vi "F5xxx Config Panel.vi"(8 "error in":errorcluster, 11 "session in":T2) -> (0 "error out":errorcluster, 3 "session out":T2)   [LabVIEW 2020]
doc: "Fluke 5000 series calibrators configuration panel."
uses:
  F5xxx_session.ctl
  F5xxx_output_mode.ctl
  <vilib>/Utility/error.llb/DialogType.ctl
panel:
  in  "btn test":bool caption="OK Button"
  out "idn string":string caption="Identification string"
  in  "btn ok":bool caption="OK Button"
  in  "ext ref clk":bool
  in  "earth":bool
  in  "mode":T1 caption="Output mode"
  in  "VISA":refnum<visa-resource-name> caption="VISA address"
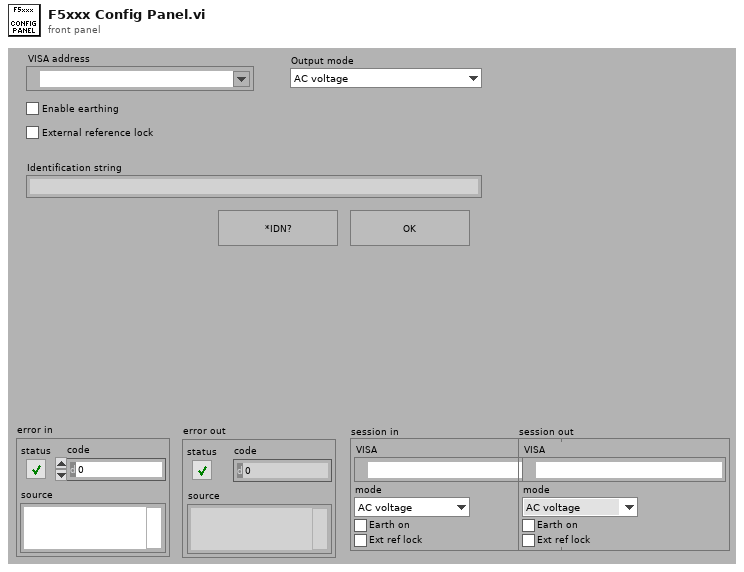
[diagram p1: front panel]
types:
  T1 = typedef "F5xxx_output_mode.ctl" = enum16{"AC voltage", "AC current"}
  T2 = typedef "F5xxx_session.ctl" = cluster{"VISA":refnum<visa-resource-name>, "mode":T1, "Earth on":bool, "Ext ref lock":bool}
  T3 = typedef "DialogType.ctl" = u16
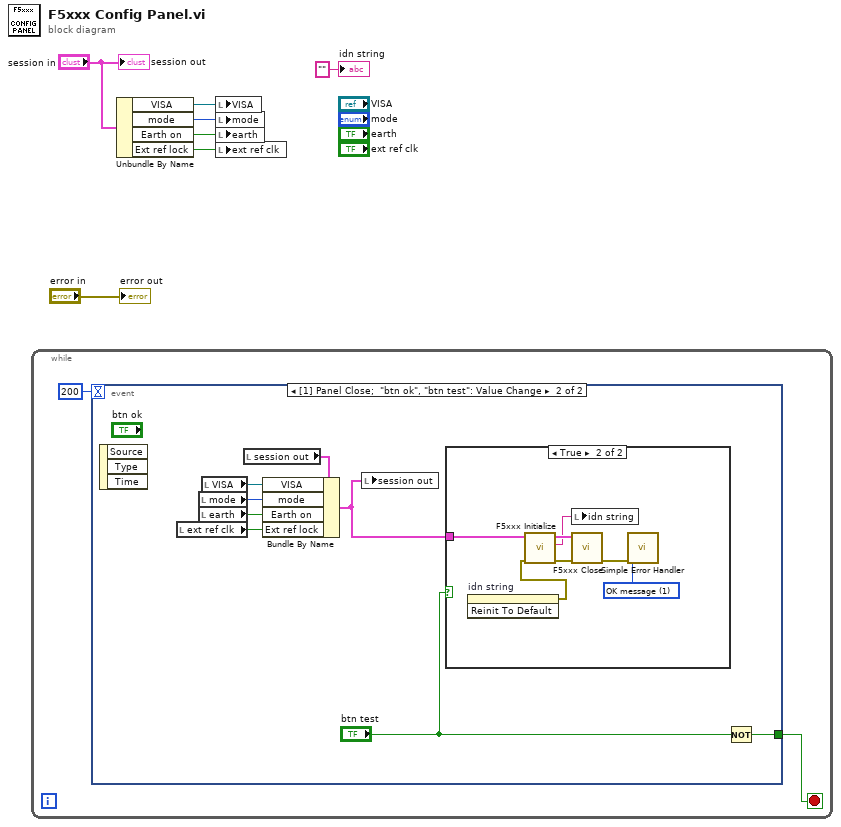
[diagram p0: block diagram]
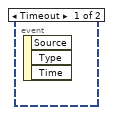
[diagram p2: hidden frame]
diagram:
  n1 = while {
    stop <- w9 stop-if-true
    n2 = event shown="[1] Panel Close;  \"btn ok\", \"btn test\": Value Change" {
      selector: _ -> [_ _]
      dyn-events: _ -> [_ _]
      timeout: 200 -> [_ _]
      tunnel: [_ w12] -> w9
      event Timeout {
        n3 = event-data() -> ()  [unwired: 1 in, 3 out]
      }
      event Panel Close; "btn ok", "btn test": Value Change {
        n4 = event-data() -> ()  [unwired: 1 in, 3 out]
        n5 = local read "ext ref clk"() -> (w13:bool)
        n6 = local read "mode"() -> (w15:T1)
        n7 = local read "earth"() -> (w14:bool)
        n8 = local read "VISA"() -> (w16:refnum<visa-resource-name>)
        n9 = local read "session out"() -> (w17:T2)
        n10 = Bundle By Name(cluster=w17, "VISA"=w16, "mode"=w15, "Earth on"=w14, "Ext ref lock"=w13) -> (w11:T2)
        n11 = local write "session out"(w11) -> ()
        n12 = case shown="True" "btn test" {
          tunnel: w11 -> [_ w24]
          frame False {
          }
          frame True {
            w20 = T3 1 items=["no dialog", "OK message", "continue or stop message", "OK message + warnings", "continue/stop + warnings"] ("type of dialog (OK msg:1)")
            n13 = invoke on="idn string" class="Str" method="Reinit To Default"() -> (error out=w19:errorcluster)  [unwired: 3 in, 2 out]
            n14 = call "F5xxx Initialize.vi"("error in (no error)"=w19, "session in"=w24) -> ("error out"=w23:errorcluster, "idn string"=w18:string, "session out"=w22:T2)  [unwired: 7 in]
            n15 = local write "idn string"(w18) -> ()
            n16 = call "F5xxx Close.vi"("error in (no error)"=w23, "session in"=w22) -> ("error out"=w21:errorcluster)  [unwired: 8 in, 1 out]
            n17 = call <vilib>:"Simple Error Handler.vi"("type of dialog (OK msg:1)"=w20, "error in (no error)"=w21) -> ()  [unwired: 3 in, 5 out]
          }
        }
        n18 = Not(x="btn test") -> (.not. x?=w12:bool)
      }
    }
  }
  n19 = Unbundle By Name("session in") -> ("VISA"=w5:refnum<visa-resource-name>, "mode"=w4:T1, "Earth on"=w3:bool, "Ext ref lock"=w2:bool)
  n20 = local write "VISA"(w5) -> ()
  n21 = local write "mode"(w4) -> ()
  n22 = local write "earth"(w3) -> ()
  n23 = local write "ext ref clk"(w2) -> ()
  "error out" <- "error in"
  "session out" <- "session in"
  "idn string" <- "" ("idn string")
